vi "Vision VI.vi"(0 "Image In":T1, 7 "error in":errorcluster) -> (20 "Image Out":T1, 25 "Particle Measurements (Pixels)[0]":dbl, 27 "error out":errorcluster)   [LabVIEW 2014]
uses:
  <vilib>/vision/Image Controls.llb/IMAQ Image.ctl
  <vilib>/vision/NI_Vision_Development_Module.lvlib
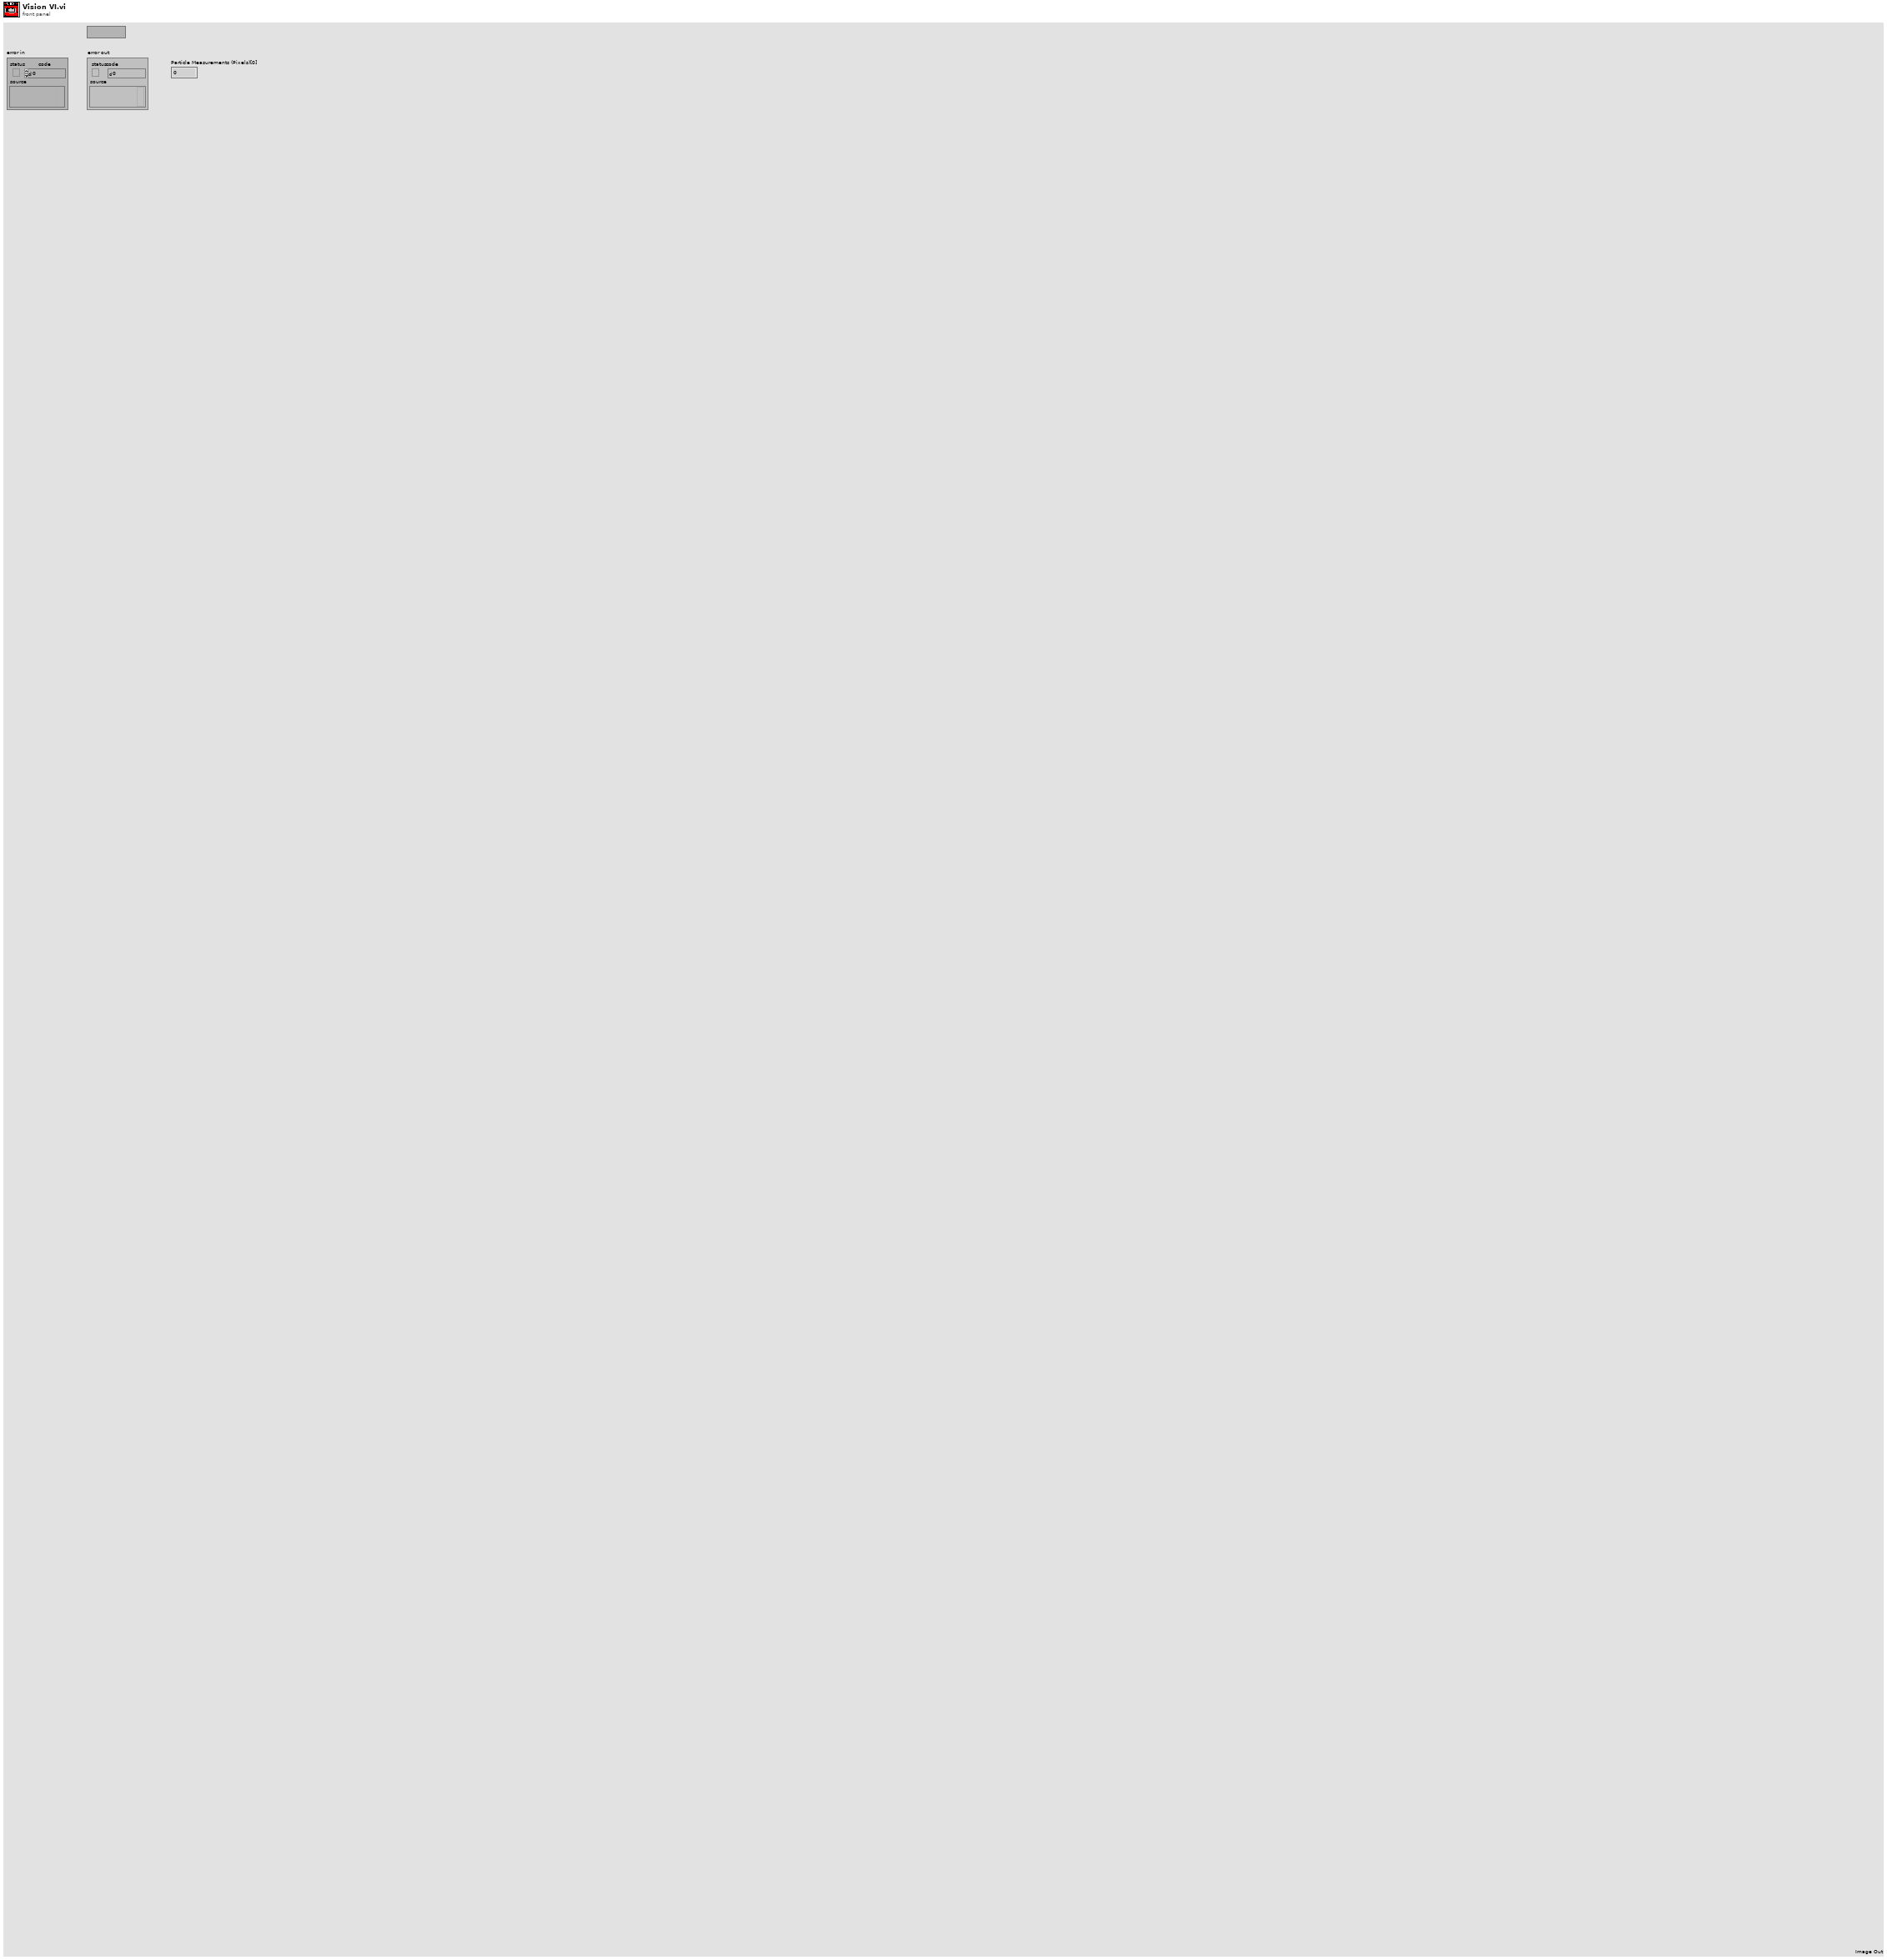
[diagram p1: front panel]
types:
  T1 = typedef "IMAQ Image.ctl" = refnum<image>
  T2 = enum32{"AutoM", "Close", "Dilate", "Erode", "Gradient", "Gradient out", "Gradient in", "Hit miss", "Open", "PClose", "POpen", "Thick", "Thin"}
  T3 = enum32{"AutoM", "Close", "Dilate", "Erode", "Gradient", "Gradient in", "Gradient out", "HitMiss", "Open", "PClose", "POpen", "Thick", "Thin"}
  T4 = cluster{"Brightness":sgl, "Contrast":sgl, "Gamma":sgl}
  T5 = cluster{"Particle Measurements (Pixels)[0]":dbl, "Particle Measurements (Pixels)[1]":dbl, "Particle Measurements (Pixels)[2]":dbl, "Particle Measurements (Pixels)[3]":dbl, "Particle Measurements (Pixels)[4]":dbl, "Particle Measurements (Pixels)[5]":dbl, "Particle Measurements (Pixels)[6]":dbl, "Particle Measurements (Pixels)[7]":dbl, "Particle Measurements (Pixels)[8]":dbl}
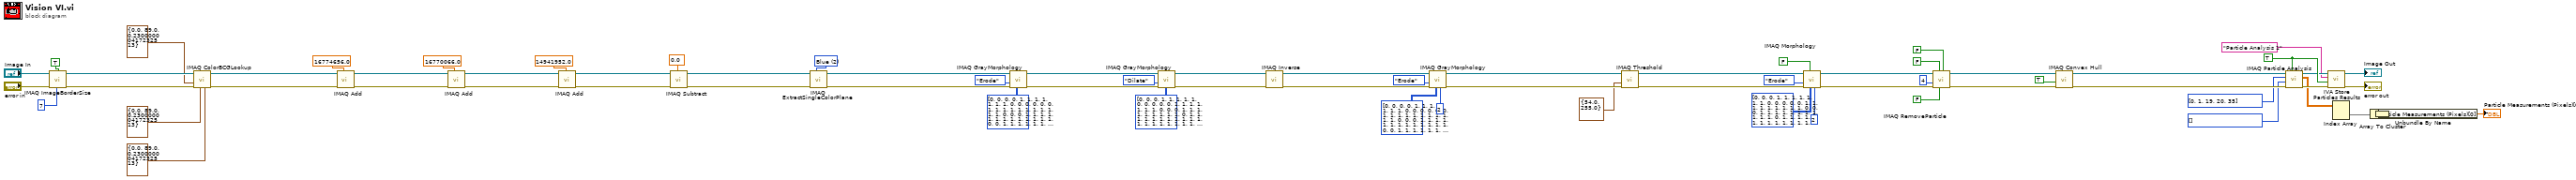
[diagram p0: block diagram]
diagram:
  w12 = i32[] [] items=["Center of Mass X", "Center of Mass Y", "First Pixel X", "First Pixel Y", "Bounding Rect Left", "Bounding Rect Top", "Bounding Rect Right", "Bounding Rect Bottom", "Max Feret Diameter Start X", "Max Feret Diameter Start Y", "Max Feret Diameter End X", "Max Feret Diameter End Y", "Max Horiz. Segment Length Left", "Max Horiz. Segment Length Right", "Max Horiz. Segment Length Row", "-", "Bounding Rect Width", "Bounding Rect Height", "Bounding Rect Diagonal", "Perimeter", "Convex Hull Perimeter", "Holes' Perimeter", "Max Feret Diameter", "Equivalent Ellipse Major Axis", "Equivalent Ellipse Minor Axis", "Equivalent Ellipse Minor Axis (Feret)", "Equivalent Rect Long Side", "Equivalent Rect Short Side", "Equivalent Rect Diagonal", "Equivalent Rect Short Side (Feret)", "Average Horiz. Segment Length", "Average Vert. Segment Length", "Hydraulic Radius", "Waddel Disk Diameter", "-", "Area", "Holes' Area", "Particle & Holes' Area", "Convex Hull Area", "Image Area", "-", "Number of Holes", "Number of Horiz. Segments", "Number of Vert. Segments", "-", "Orientation", "Max Feret Diameter Orientation", "-", "% Area/Image Area", "% Area/(Particle & Holes' Area)", "Ratio of Equivalent Ellipse Axes", "Ratio of Equivalent Rect Sides", "-", "Elongation Factor", "Compactness Factor", "Heywood Circularity Factor", "Type Factor", "-", "Sum X", "Sum Y", "Sum XX", "Sum XY", "Sum YY", "Sum XXX", "Sum XXY", "Sum XYY", "Sum YYY", "-", "Moment of Inertia XX", "Moment of Inertia XY", "Moment of Inertia YY", "Moment of Inertia XXX", "Moment of Inertia XXY", "Moment of Inertia XYY", "Moment of Inertia YYY", "Norm. Moment of Inertia XX", "Norm. Moment of Inertia XY", "Norm. Moment of Inertia YY", "Norm. Moment of Inertia XXX", "Norm. Moment of Inertia XXY", "Norm. Moment of Inertia XYY", "Norm. Moment of Inertia YYY", "Hu Moment 1", "Hu Moment 2", "Hu Moment 3", "Hu Moment 4", "Hu Moment 5", "Hu Moment 6", "Hu Moment 7"] ("Real-World Measurements")
  w13 = i32[] [0, 1, 19, 20, 35] items=["Center of Mass X", "Center of Mass Y", "First Pixel X", "First Pixel Y", "Bounding Rect Left", "Bounding Rect Top", "Bounding Rect Right", "Bounding Rect Bottom", "Max Feret Diameter Start X", "Max Feret Diameter Start Y", "Max Feret Diameter End X", "Max Feret Diameter End Y", "Max Horiz. Segment Length Left", "Max Horiz. Segment Length Right", "Max Horiz. Segment Length Row", "-", "Bounding Rect Width", "Bounding Rect Height", "Bounding Rect Diagonal", "Perimeter", "Convex Hull Perimeter", "Holes' Perimeter", "Max Feret Diameter", "Equivalent Ellipse Major Axis", "Equivalent Ellipse Minor Axis", "Equivalent Ellipse Minor Axis (Feret)", "Equivalent Rect Long Side", "Equivalent Rect Short Side", "Equivalent Rect Diagonal", "Equivalent Rect Short Side (Feret)", "Average Horiz. Segment Length", "Average Vert. Segment Length", "Hydraulic Radius", "Waddel Disk Diameter", "-", "Area", "Holes' Area", "Particle & Holes' Area", "Convex Hull Area", "Image Area", "-", "Number of Holes", "Number of Horiz. Segments", "Number of Vert. Segments", "-", "Orientation", "Max Feret Diameter Orientation", "-", "% Area/Image Area", "% Area/(Particle & Holes' Area)", "Ratio of Equivalent Ellipse Axes", "Ratio of Equivalent Rect Sides", "-", "Elongation Factor", "Compactness Factor", "Heywood Circularity Factor", "Type Factor", "-", "Sum X", "Sum Y", "Sum XX", "Sum XY", "Sum YY", "Sum XXX", "Sum XXY", "Sum XYY", "Sum YYY", "-", "Moment of Inertia XX", "Moment of Inertia XY", "Moment of Inertia YY", "Moment of Inertia XXX", "Moment of Inertia XXY", "Moment of Inertia XYY", "Moment of Inertia YYY", "Norm. Moment of Inertia XX", "Norm. Moment of Inertia XY", "Norm. Moment of Inertia YY", "Norm. Moment of Inertia XXX", "Norm. Moment of Inertia XXY", "Norm. Moment of Inertia XYY", "Norm. Moment of Inertia YYY", "Hu Moment 1", "Hu Moment 2", "Hu Moment 3", "Hu Moment 4", "Hu Moment 5", "Hu Moment 6", "Hu Moment 7"] ("Pixel Measurements")
  w10 = TRUE ("Connectivity 4/8 (8)")
  w49 = 2 items=["Red", "Green", "Blue", "Hue", "Saturation", "Luminance", "Value", "Intensity"] ("Color Plane")
  n1 = call "IMAQ ImageBorderSize"("Get/Set Status? (Set)"=TRUE, "Image"="Image In", "Image border size in"=7 ("Border Size"), "error in (no error)"="error in") -> ("Image Out"=w66:T1, "error out"=w69:errorcluster)  [unwired: 1 out]
  n2 = call "IMAQ ColorBCGLookup"("Blue BCG Values"=T4 {"Brightness"=0.0, "Contrast"=89.0, "Gamma"=0.23}, "Green BCG Values"=T4 {"Brightness"=0.0, "Contrast"=89.0, "Gamma"=0.23}, "error in (no error)"=w69, "Red BCG Values"=T4 {"Brightness"=0.0, "Contrast"=89.0, "Gamma"=0.23}, "Image Src"=w66) -> ("error out"=w65:errorcluster, "Image Dst Out"=w60:T1)  [unwired: 2 in, 3 out]
  n3 = call "IMAQ Add"("Image Src A"=w60, "Constant"=sgl 16774656.0, "error in (no error)"=w65) -> ("Image Dst Out"=w57:T1, "error out"=w59:errorcluster)  [unwired: 2 in, 2 out]
  n4 = call "IMAQ Add"("Image Src A"=w57, "Constant"=sgl 16770066.0, "error in (no error)"=w59) -> ("Image Dst Out"=w54:T1, "error out"=w56:errorcluster)  [unwired: 2 in, 2 out]
  n5 = call "IMAQ Add"("Image Src A"=w54, "Constant"=sgl 14941952.0, "error in (no error)"=w56) -> ("Image Dst Out"=w51:T1, "error out"=w53:errorcluster)  [unwired: 2 in, 2 out]
  n6 = call "IMAQ Subtract"("Image Src A"=w51, "Constant"=sgl 0.0, "error in (no error)"=w53) -> ("Image Dst Out"=w48:T1, "error out"=w50:errorcluster)  [unwired: 2 in, 2 out]
  n7 = call "IMAQ ExtractSingleColorPlane"("Color Plane"=w49, "error in (no error)"=w50, "Image Src"=w48) -> ("error out"=w47:errorcluster, "Image Dst Out"=w44:T1)  [unwired: 1 in, 6 out]
  n8 = call "IMAQ GrayMorphology"("Structuring Element"=i32[][] [[0, 0, 0, 0, 1, 1, 1, 1, 1, 1, 1, 0, 0, 0, 0], [0, 0, 1, 1, 1, 1, 1, 1, 1, 1, 1, 1, 1, 0, 0], [0, 1, 1, 1, 1, 1, 1, 1, 1, 1, 1, 1, 1, 1, 0], [0, 1, 1, 1, 1, 1, 1, 1, 1, 1, 1, 1, 1, 1, 0], [1, 1, 1, 1, 1, 1, 1, 1, 1, 1, 1, 1, 1, 1, 1], [1, 1, 1, 1, 1, 1, 1, 1, 1, 1, 1, 1, 1, 1, 1], [1, 1, 1, 1, 1, 1, 1, 1, 1, 1, 1, 1, 1, 1, 1], [1, 1, 1, 1, 1, 1, 1, 1, 1, 1, 1, 1, 1, 1, 1], [1, 1, 1, 1, 1, 1, 1, 1, 1, 1, 1, 1, 1, 1, 1], [1, 1, 1, 1, 1, 1, 1, 1, 1, 1, 1, 1, 1, 1, 1], [1, 1, 1, 1, 1, 1, 1, 1, 1, 1, 1, 1, 1, 1, 1], [0, 1, 1, 1, 1, 1, 1, 1, 1, 1, 1, 1, 1, 1, 0], [0, 1, 1, 1, 1, 1, 1, 1, 1, 1, 1, 1, 1, 1, 0], [0, 0, 1, 1, 1, 1, 1, 1, 1, 1, 1, 1, 1, 0, 0], [0, 0, 0, 0, 1, 1, 1, 1, 1, 1, 1, 0, 0, 0, 0]], "error in (no error)"=w47, "Operation"=T3."Erode", "Image Src"=w44) -> ("error out"=w43:errorcluster, "Image Dst Out"=w40:T1)  [unwired: 3 in, 3 out]
  n9 = call "IMAQ GrayMorphology"("Structuring Element"=i32[][] [[0, 0, 0, 1, 1, 1, 1, 1, 0, 0, 0], [0, 0, 1, 1, 1, 1, 1, 1, 1, 0, 0], [0, 1, 1, 1, 1, 1, 1, 1, 1, 1, 0], [1, 1, 1, 1, 1, 1, 1, 1, 1, 1, 1], [1, 1, 1, 1, 1, 1, 1, 1, 1, 1, 1], [1, 1, 1, 1, 1, 1, 1, 1, 1, 1, 1], [1, 1, 1, 1, 1, 1, 1, 1, 1, 1, 1], [1, 1, 1, 1, 1, 1, 1, 1, 1, 1, 1], [0, 1, 1, 1, 1, 1, 1, 1, 1, 1, 0], [0, 0, 1, 1, 1, 1, 1, 1, 1, 0, 0], [0, 0, 0, 1, 1, 1, 1, 1, 0, 0, 0]], "error in (no error)"=w43, "Operation"=T3."Dilate", "Image Src"=w40) -> ("error out"=w39:errorcluster, "Image Dst Out"=w38:T1)  [unwired: 3 in, 3 out]
  n10 = call "IMAQ Inverse"("error in (no error)"=w39, "Image Src"=w38) -> ("error out"=w37:errorcluster, "Image Dst Out"=w34:T1)  [unwired: 2 in, 6 out]
  n11 = call "IMAQ GrayMorphology"("Number of iterations (1)"=2, "Structuring Element"=i32[][] [[0, 0, 0, 0, 1, 1, 1, 1, 1, 1, 1, 0, 0, 0, 0], [0, 0, 1, 1, 1, 1, 1, 1, 1, 1, 1, 1, 1, 0, 0], [0, 1, 1, 1, 1, 1, 1, 1, 1, 1, 1, 1, 1, 1, 0], [0, 1, 1, 1, 1, 1, 1, 1, 1, 1, 1, 1, 1, 1, 0], [1, 1, 1, 1, 1, 1, 1, 1, 1, 1, 1, 1, 1, 1, 1], [1, 1, 1, 1, 1, 1, 1, 1, 1, 1, 1, 1, 1, 1, 1], [1, 1, 1, 1, 1, 1, 1, 1, 1, 1, 1, 1, 1, 1, 1], [1, 1, 1, 1, 1, 1, 1, 1, 1, 1, 1, 1, 1, 1, 1], [1, 1, 1, 1, 1, 1, 1, 1, 1, 1, 1, 1, 1, 1, 1], [1, 1, 1, 1, 1, 1, 1, 1, 1, 1, 1, 1, 1, 1, 1], [1, 1, 1, 1, 1, 1, 1, 1, 1, 1, 1, 1, 1, 1, 1], [0, 1, 1, 1, 1, 1, 1, 1, 1, 1, 1, 1, 1, 1, 0], [0, 1, 1, 1, 1, 1, 1, 1, 1, 1, 1, 1, 1, 1, 0], [0, 0, 1, 1, 1, 1, 1, 1, 1, 1, 1, 1, 1, 0, 0], [0, 0, 0, 0, 1, 1, 1, 1, 1, 1, 1, 0, 0, 0, 0]], "error in (no error)"=w37, "Operation"=T3."Erode", "Image Src"=w34) -> ("error out"=w33:errorcluster, "Image Dst Out"=w30:T1)  [unwired: 2 in, 3 out]
  n12 = call "IMAQ Threshold"("error in (no error)"=w33, "Range"=cluster{"Lower value":sgl, "Upper value":sgl} {"Lower value"=54.0, "Upper value"=255.0}, "Image Src"=w30) -> ("error out"=w29:errorcluster, "Image Dst Out"=w24:T1)  [unwired: 3 in, 4 out]
  n13 = call "IMAQ Morphology"("Number of iterations (1)"=2, "Structuring Element"=i32[][] [[0, 0, 0, 1, 1, 1, 1, 1, 1, 1, 0, 0, 0], [0, 0, 1, 1, 1, 1, 1, 1, 1, 1, 1, 0, 0], [0, 1, 1, 1, 1, 1, 1, 1, 1, 1, 1, 1, 0], [1, 1, 1, 1, 1, 1, 1, 1, 1, 1, 1, 1, 1], [1, 1, 1, 1, 1, 1, 1, 1, 1, 1, 1, 1, 1], [1, 1, 1, 1, 1, 1, 1, 1, 1, 1, 1, 1, 1], [1, 1, 1, 1, 1, 1, 1, 1, 1, 1, 1, 1, 1], [1, 1, 1, 1, 1, 1, 1, 1, 1, 1, 1, 1, 1], [1, 1, 1, 1, 1, 1, 1, 1, 1, 1, 1, 1, 1], [1, 1, 1, 1, 1, 1, 1, 1, 1, 1, 1, 1, 1], [0, 1, 1, 1, 1, 1, 1, 1, 1, 1, 1, 1, 0], [0, 0, 1, 1, 1, 1, 1, 1, 1, 1, 1, 0, 0], [0, 0, 0, 1, 1, 1, 1, 1, 1, 1, 0, 0, 0]], "Square/Hexa (Square)"=FALSE, "error in (no error)"=w29, "Operation"=T2."Erode", "Image Src"=w24) -> ("error out"=w23:errorcluster, "Image Dst Out"=w18:T1)  [unwired: 1 in, 3 out]
  n14 = call "IMAQ RemoveParticle"("Connectivity 4/8 (8)"=FALSE, "Low Pass/High Pass (Low)"=FALSE, "Square/Hexa (Square)"=FALSE, "error in (no error)"=w23, "Number of Erosion"=4, "Image Src"=w18) -> ("error out"=w17:errorcluster, "Image Dst Out"=w16:T1)  [unwired: 1 in, 3 out]
  n15 = call "IMAQ Convex Hull"("error in (no error)"=w17, "Connectivity 4/8 (8)"=TRUE, "Image Src"=w16) -> ("error out"=w14:errorcluster, "Image Dst Out"=w11:T1)  [unwired: 1 in, 6 out]
  n16 = call "IMAQ Particle Analysis"("Connectivity 4/8 (8)"=w10, "error in (no error)"=w14, "Real-World Measurements"=w12, "Pixel Measurements"=w13, "Image"=w11) -> ("error out"=w6:errorcluster, "Particle Measurements (Pixels)"=w2:dbl[][], "Image Out (duplicate)"=w9:T1)  [unwired: 4 out]
  n17 = call <vilib>:"IVA Store Particles Results.vi"("error in (no error)"=w6, "Connectivity 4/8 (8)"=w10, "Step Name"="Particle Analysis 1", "Image in"=w9) -> ("error out"=→"error out":errorcluster, "Image dup"=→"Image Out":T1)  [unwired: 6 out]
  n18 = Index Array(array=w2) -> (element=w4:dbl[])  [unwired: 2 in]
  n19 = Array To Cluster(array=w4) -> (cluster=w3:T5)
  n20 = Unbundle By Name(w3) -> ("Particle Measurements (Pixels)[0]"=→"Particle Measurements (Pixels)[0]":dbl)
